vi "Simulated Temperature Control.vi"() -> ()   [LabVIEW 2010]
uses:
  SupportVIs.llb/TS_RT-globalvar.vi
  SupportVIs.llb/TS_RT-Integrator (DBL).vi
  SupportVIs.llb/TS_RT-PID (DBL).vi
panel:
  out "Stabilized":bool
  in  "stop":bool
  out "Temperature":dbl(slide) scale=0.0..100.0
  in  "Setpoint":dbl=20.0 format="%.2f"
  in  "PID gains":T1={"proportional gain (Kc)"=1.0, "integral time (Ti, min)"=2.0, "derivative time (Td, min)"=0.0} {"derivative time (Td, min)" format="%.3f"; "integral time (Ti, min)" format="%.3f"; "proportional gain (Kc)" format="%.3f"}
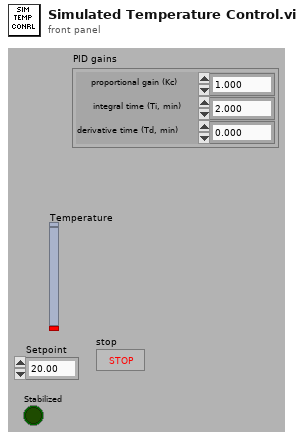
[diagram p1: front panel]
types:
  T1 = cluster{"proportional gain (Kc)":dbl, "integral time (Ti, min)":dbl, "derivative time (Td, min)":dbl}
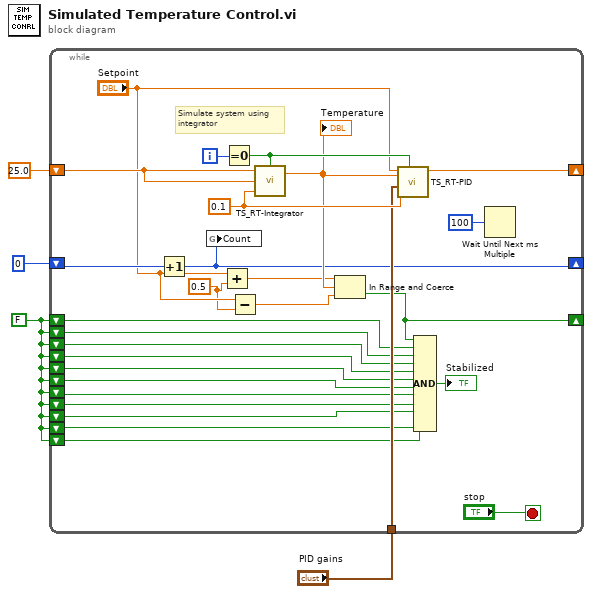
[diagram p0: block diagram]
diagram:
  w1 = FALSE
  n1 = while {
    shift-right: [w27] -> _
    shift-left: 25.0 ("output") -> [w32]
    tunnel: "PID gains" -> [w25]
    shift-right: [w9] -> _
    shift-left: 0 -> [w24]
    shift-right: [w23] -> _
    shift-left: w1 -> [w22]
    shift-left: w1 -> [w21]
    shift-left: w1 -> [w20]
    shift-left: w1 -> [w19]
    shift-left: w1 -> [w18]
    shift-left: w1 -> [w17]
    shift-left: w1 -> [w16]
    shift-left: w1 -> [w15]
    shift-left: w1 -> [w14]
    shift-left: w1 -> [w13]
    shift-left: w1 -> [w12]
    i -> [w31]
    stop <- "stop" stop-if-true
    w6 = 0.5 ("y")
    w29 = 0.1 ("dt")
    # "Simulate system using\nintegrator"
    n2 = Increment(x=w24) -> (x+1=w9:i32)
    n3 = global write "TS_RT-globalvar.vi" "Count"(w9) -> ()
    n4 = Add(x="Setpoint", y=w6) -> (x+y=w8:dbl)
    n5 = Equal To 0?(x=w31) -> (x = 0?=w28:bool)
    n6 = Subtract(x="Setpoint", y=w6) -> (x-y=w5:dbl)
    n7 = call-poly "TS_RT-Integrator.vi"("initialize"=w28, "dt"=w29, "initial condition"=w32, "input point"=w32) -> ("output point"=w10:dbl)  [unwired: 1 out]
    "Temperature" <- w10
    n8 = In Range and Coerce(upper limit=w8, x=w10, lower limit=w5) -> (In Range?=w23:bool)  [unwired: 1 out]
    n9 = call-poly "TS_RT-PID.vi"("reinitialize? (F)"=w28, "dt (s)"=w29, "PID gains"=w25, "process variable"=w10, "setpoint"="Setpoint") -> ("output"=w27:dbl)  [unwired: 1 in, 5 out]
    n10 = Compound Arithmetic op=AND(w23, w22, w21, w20, w19, w18, w17, w16, w15, w14, w13, w12) -> (→"Stabilized":bool)
    n11 = Wait Until Next ms Multiple(millisecond multiple=u32 100) -> ()  [unwired: 1 out]
  }
